vi "Value to String.vi"(8 "error in (no error)":errorcluster, 10 "Data Type":T1(ring), 11 "Value":variant) -> (0 "error out":errorcluster, 3 "Value String":string)   [LabVIEW 2024]
doc: "Converts variant data to a string."
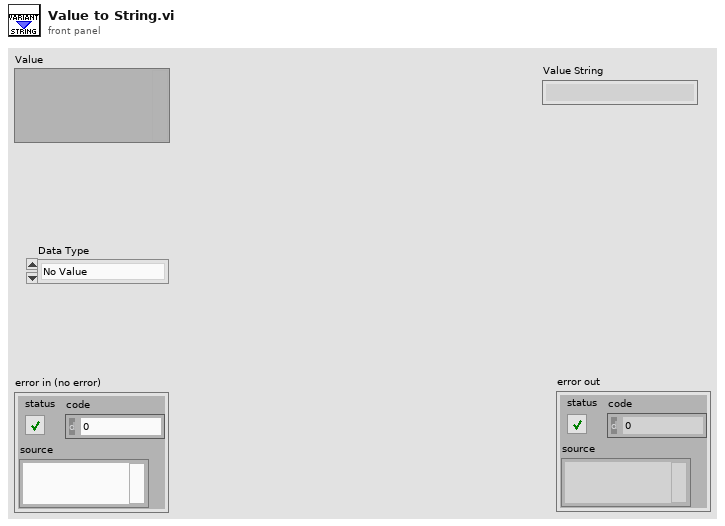
[diagram p1: front panel]
types:
  T1 = enum16{"No Value", "Custom", "Double", "Boolean", "U32", "String", "DBL Array", "I32 Array", "I32", "SGL Array", "SGL", "I8", "U8", "I16", "U16", "I64", "U64", "DBL Waveform", "I16 Waveform", "Boolean Array", "I8 Array", "U8 Array", "I16 Array", "U16 Array", "U32 Array", "I64 Array", "U64 Array", "DBL Waveform Array", "I16 Waveform Array"}
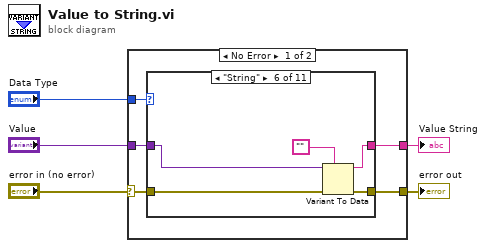
[diagram p0: block diagram]
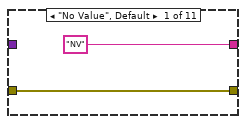
[diagram p2: hidden frame]
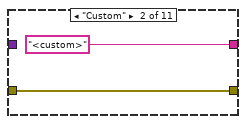
[diagram p3: hidden frame]
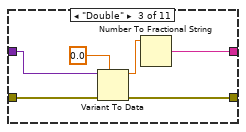
[diagram p4: hidden frame]
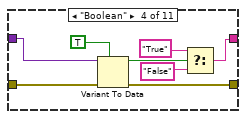
[diagram p5: hidden frame]
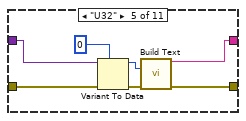
[diagram p6: hidden frame]
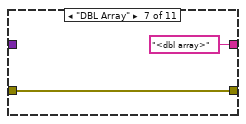
[diagram p7: hidden frame]
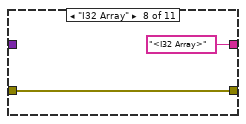
[diagram p8: hidden frame]
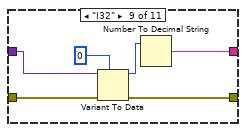
[diagram p9: hidden frame]
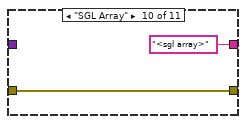
[diagram p10: hidden frame]
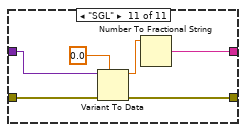
[diagram p11: hidden frame]
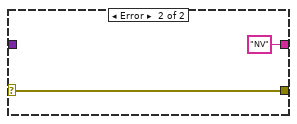
[diagram p12: hidden frame]
diagram:
  n1 = case shown="No Error" "error in (no error)" {
    selector: "error in (no error)" -> [w6 w60]
    tunnel: [w7 w60] -> w4
    tunnel: [w10 "NV"] -> w3
    tunnel: "Value" -> [w9 _]
    tunnel: "Data Type" -> [w8 _]
    frame No Error {
      n2 = case shown="\"String\"" w8 {
        tunnel: w9 -> [_ _ w20 w28 w35 w40 _ _ w50 _ w55]
        tunnel: ["NV" "<custom>" w17 w23 w32 w38 "<dbl array>" ("Result") "<I32 Array>" ("Result") w47 "<sgl array>" ("Result") w56] -> w10
        tunnel: [w11 w13 w16 w22 w30 w36 w41 w43 w45 w51 w53] -> w7
        tunnel: w6 -> [w11 w13 w15 w21 w29 w37 w41 w43 w46 w51 w54]
        frame "No Value", Default {
        }
        frame "Custom" {
        }
        frame "Double" {
          n3 = Variant To Data(error in=w15, type=0.0 ("disabled index (col)"), Variant=w20) -> (data=w18:dbl, error out=w16:errorcluster)
          n4 = Number To Fractional String(number=w18) -> (F-format string=w17:string)  [unwired: 3 out]
        }
        frame "Boolean" {
          n5 = Variant To Data(error in=w21, type=TRUE, Variant=w28) -> (data=w26:bool, error out=w22:errorcluster)
          n6 = Select(t="True", s=w26, f="False") -> (s? t:f=w23:string)
        }
        frame "U32" {
          n7 = Variant To Data(error in=w29, type=u32 0, Variant=w35) -> (data=w33:u32, error out=w31:errorcluster)
          n8 = call "Build Text"("bitarray"=w33, "error in (no error)"=w31) -> ("Result"=w32:string, "error out"=w30:errorcluster)  [unwired: 1 in, 11 out]
        }
        frame "String" {
          n9 = Variant To Data(error in=w37, type="", Variant=w40) -> (data=w38:string, error out=w36:errorcluster)
        }
        frame "DBL Array" {
        }
        frame "I32 Array" {
        }
        frame "I32" {
          n10 = Variant To Data(error in=w46, type=0 ("disabled index (row)"), Variant=w50) -> (data=w48:i32, error out=w45:errorcluster)
          n11 = Number To Decimal String(number=w48) -> (decimal integer string=w47:string)  [unwired: 1 out]
        }
        frame "SGL Array" {
        }
        frame "SGL" {
          n12 = Variant To Data(error in=w54, type=sgl 0.0 ("disabled index (col)"), Variant=w55) -> (data=w57:sgl, error out=w53:errorcluster)
          n13 = Number To Fractional String(number=w57) -> (F-format string=w56:string)  [unwired: 3 out]
        }
      }
    }
    frame Error {
    }
  }
  "error out" <- w4
  "Value String" <- w3
